vi "信息转换.vi"(8 "错误输入（无错误）":errorcluster, 10 "追溯码":string[](array[string]), 11 "测试信息":T1) -> (0 "错误输出":errorcluster, 3 "信息输出":string[](array[string]))   [LabVIEW 2020]
uses:
  <vilib>/addons/database/Connection.llb/DB Tools Open Connec (String).vi
  <vilib>/addons/database/Connection.llb/Conn Execute.vi
  <vilib>/addons/database/Recordset.llb/Rec Fetch Recordset Data (R).vi
  <vilib>/addons/database/Recordset.llb/Rec Destroy - Connection.vi
  <vilib>/addons/database/NI_Database_API.lvlib
panel:
  out "error out":errorcluster
  in  "error in (no error)":errorcluster caption="错误输入（无错误）"
  # "用户信息转换"
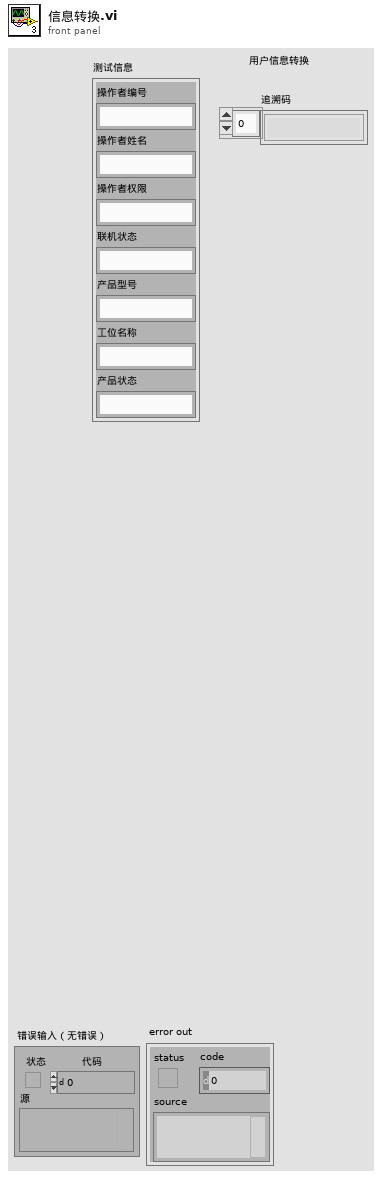
[diagram p1: front panel]
types:
  T1 = cluster{"操作者编号":string, "操作者姓名":string, "操作者权限":string, "联机状态":string, "产品型号":string, "工位名称":string, "产品状态":string}
  T2 = typedef "NI_Database_API.lvlib/Conn ObjectReference.ctl" = refnum<k1>
  T3 = typedef "NI_Database_API.lvlib/Rec ObjectReference.ctl" = refnum<k1>
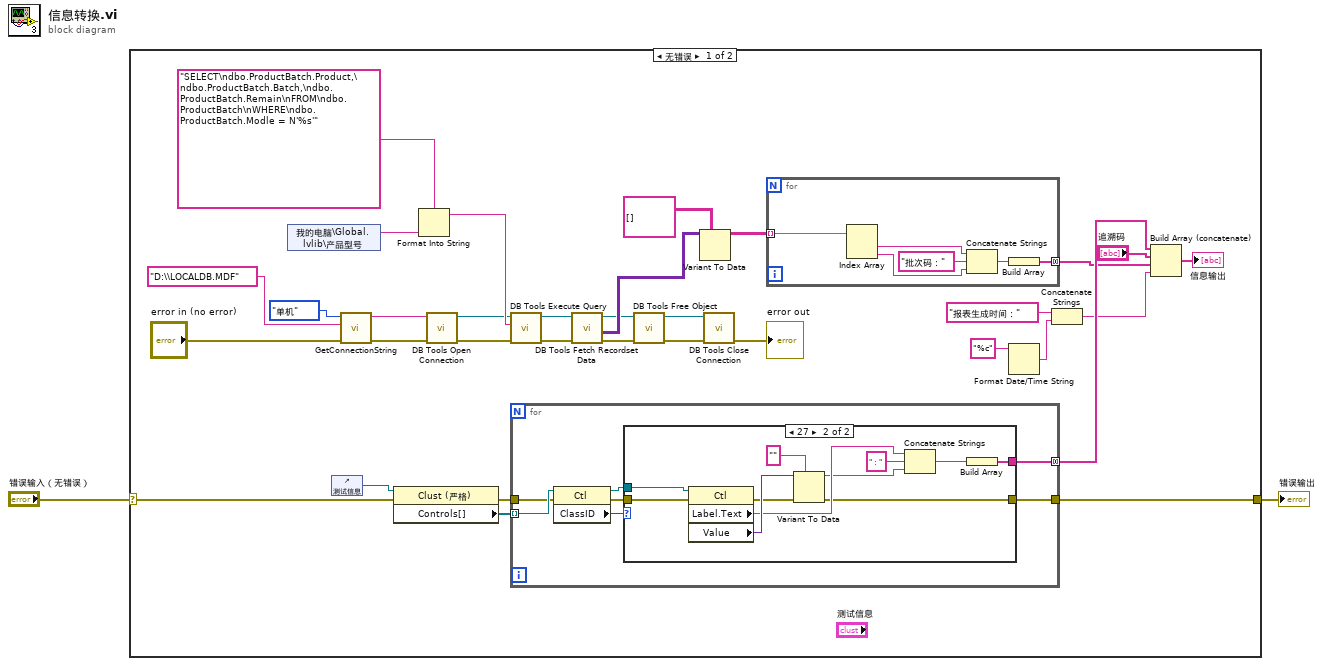
[diagram p0: block diagram]
diagram:
  n1 = case shown="无错误" "错误输入（无错误）" {
    selector: "错误输入（无错误）" -> [w28 w61]
    tunnel: [w26 w61] -> w1
    frame No Error {
      n2 = shared-variable "我的电脑\\Global.lvlib\\产品型号"() -> (w3:string)  [unwired: 1 in, 1 out]
      n3 = control-ref of="测试信息"() -> (w35:refnum<vi>)
      n4 = call "GetConnectionString.vi"("error in (no error)"="error in (no error)", "Database Name"="D:\\LOCALDB.MDF", "连接模式"=enum16{"单机", "联网"}."单机") -> ("error out"=w8:errorcluster, "连接字符串"=w9:string)  [unwired: 3 in]
      n5 = property on="属性节点" class="Clust (严格)"(reference=w35, error in=w28) -> (error out=w27:errorcluster, "Controls[]"=w34:refnum<vi>[])  [unwired: 1 out]
      n6 = Format Into String(format string="SELECT\ndbo.ProductBatch.Product,\ndbo.ProductBatch.Batch,\ndbo.ProductBatch.Remain\nFROM\ndbo.ProductBatch\nWHERE\ndbo.ProductBatch.Modle = N'%s'" ("SQL query"), w3) -> (resulting string=w18:string)  [unwired: 2 in, 1 out]
      n7 = call-poly <vilib>:"DB Tools Open Connection.vi"("error in (no error)"=w8, "connection information"=w9) -> ("error out"=w10:errorcluster, "connection reference"=w11:T2)  [unwired: 6 in]
      n8 = call-poly <vilib>:"DB Tools Execute Query.vi"("error in (no error)"=w10, "SQL query"=w18, "connection reference"=w11) -> ("error out"=w12:errorcluster, "recordset reference"=w13:T3)  [unwired: 5 in]
      n9 = for {
        tunnel: w34 -> [w48] mode=indexing
        tunnel: [w45] -> w32 mode=concatenating
        tunnel: w27 -> [w44]
        tunnel: [w42] -> w26
        n10 = property class="Ctl"(reference=w48, error in=w44) -> (reference out=w46:refnum<vi>, error out=w43:errorcluster, "ClassID"=w47:u32)
        n11 = case shown="27" w47 {
          tunnel: w46 -> [_ w60]
          tunnel: [_ w53] -> w45
          tunnel: w43 -> [w49 w52]
          tunnel: [w49 w50] -> w42
          frame 0, Default {
          }
          frame 27 {
            n12 = property class="Ctl"(reference=w60, error in=w52) -> (error out=w51:errorcluster, "Label.Text"=w57:string, "Value"=w58:variant)  [unwired: 1 out]
            n13 = Variant To Data(error in=w51, type="", Variant=w58) -> (data=w56:string, error out=w50:errorcluster)
            n14 = Concatenate Strings(w57, "：" ("字符串"), w56) -> (w54:string)
            n15 = Build Array(w54) -> (w53:string[])
          }
        }
      }
      n16 = call-poly <vilib>:"DB Tools Fetch Recordset Data.vi"("error in (no error)"=w12, "recordset reference"=w13) -> ("error out"=w15:errorcluster, "recordset data"=w20:variant[][], "recordset reference out"=w14:T3)  [unwired: 3 in]
      n17 = call-poly <vilib>:"DB Tools Free Object.vi"("error in (no error)"=w15, "recordset reference"=w14) -> ("error out"=w21:errorcluster, "connection reference"=w22:T2)  [unwired: 8 in]
      n18 = Variant To Data(type=string[][] [] ("值"), Variant=w20) -> (data=w25:string[][])  [unwired: 1 in, 1 out]
      n19 = call <vilib>:"DB Tools Close Connection.vi"("error in (no error)"=w21, "connection reference"=w22) -> ("error out"=→"error out":errorcluster)  [unwired: 5 in]
      n20 = for {
        tunnel: w25 -> [w39] mode=indexing
        tunnel: [w36] -> w6 mode=concatenating
        n21 = Index Array(array=w39) -> (element #1=w38:string, element #2=w37:string)  [unwired: 2 in]
        n22 = Concatenate Strings(w38, "批次码：" ("字符串"), w37) -> (w40:string)
        n23 = Build Array(w40) -> (w36:string[])
      }
      n24 = Format Date/Time String(time format string (%c)="%c") -> (date/time string=w29:string)  [unwired: 2 in]
      n25 = Concatenate Strings("报表生成时间：" ("字符串"), w29) -> (w5:string)
      n26 = Build Array (concatenate)(w32, "追溯码", w6, w5) -> (→"信息输出":string[])
    }
    frame Error {
    }
  }
  "错误输出" <- w1
